vi "Calculate_Timescales.vi"(1 "Sampling Frequency (Hz)":dbl, 2 "Autocorrelation length":i32, 3 "Autocorrelation":dbl[](array[numeric])) -> (0 "Time Scale estimate (s)":dbl)   [LabVIEW 2011]
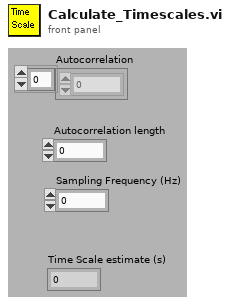
[diagram p1: front panel]
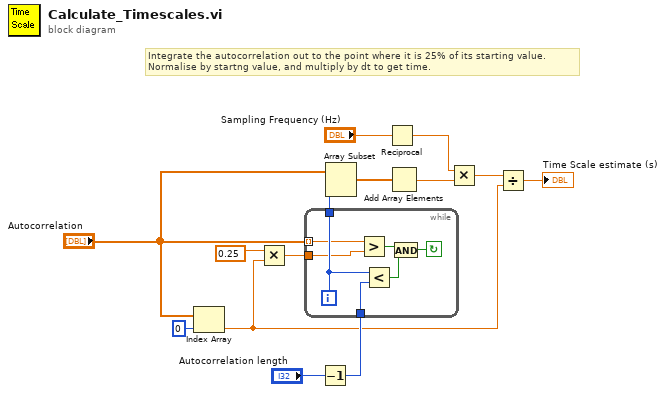
[diagram p0: block diagram]
diagram:
  # "Integrate the autocorrelation out to the point where it is 25% of its starting value.\nNormalise by startng value, and multiply by dt to get time."
  n1 = Index Array(array="Autocorrelation", index=0) -> (element=w2:dbl)
  n2 = Multiply(x=0.25 ("y"), y=w2) -> (x*y=w14:dbl)
  n3 = Decrement(x="Autocorrelation length") -> (x-1=w9:i32)
  n4 = while {
    tunnel: "Autocorrelation" -> [w15] mode=indexing
    tunnel: w9 -> [w21]
    tunnel: [w18] -> w12
    tunnel: w14 -> [w17]
    i -> [w18]
    stop <- w19 continue-if-true
    n5 = Greater?(x=w15, y=w17) -> (0:w16:bool)
    n6 = Less?(x=w18, y=w21) -> (x < y?=w20:bool)
    n7 = And(x=w16, y=w20) -> (x .and. y?=w19:bool)
  }
  n8 = Array Subset(array="Autocorrelation", length=w12) -> (w8:dbl[])  [unwired: 1 in]
  n9 = Reciprocal(x="Sampling Frequency (Hz)") -> (1/x=w4:dbl)
  n10 = Add Array Elements(numeric array=w8) -> (sum=w5:dbl)
  n11 = Multiply(x=w4, y=w5) -> (x*y=w7:dbl)
  n12 = Divide(x=w7, y=w2) -> (x/y=→"Time Scale estimate (s)":dbl)
